vi "ivPIDantiWindup_Filter.vi"(4 "Saturation U":dbl, 6 "Saturation M":dbl, 7 "Reset":bool, 8 "PID Gains":cluster{"Kp":dbl, "Kd":dbl, "Ki":dbl, "Ts":dbl}={"Kp"=0.0, "Kd"=0.0, "Ki"=0.0, "Ts"=1.0}, 10 "Feedback":dbl, 11 "Reference":dbl) -> (3 "Control":dbl)   [LabVIEW 2016]
uses:
  <vilib>/ptbypt/NI_PtbyPt.lvlib
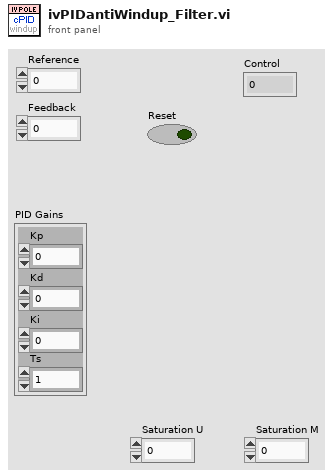
[diagram p1: front panel]
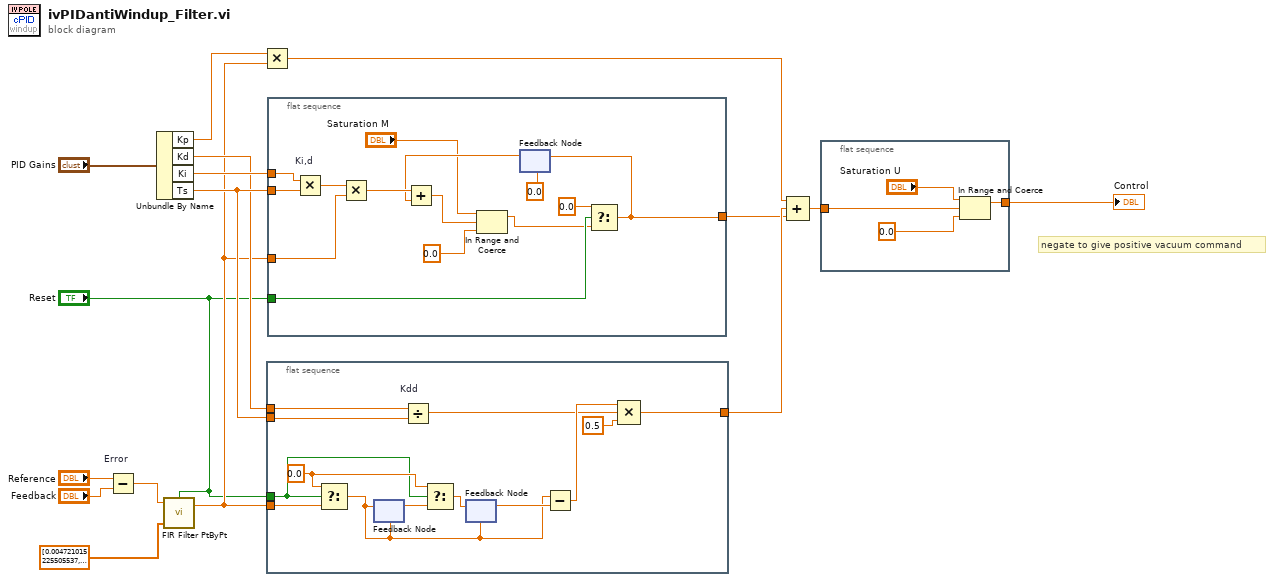
[diagram p0: block diagram]
diagram:
  # "negate to give positive vacuum command"
  n1 = Subtract "Error"(x="Reference", y="Feedback") -> (x-y=w3:dbl)
  n2 = Unbundle By Name("PID Gains") -> ("Kp"=w13:dbl, "Kd"=w7:dbl, "Ki"=w9:dbl, "Ts"=w8:dbl)
  n3 = call <vilib>:"FIR Filter PtByPt.vi"("initialize"="Reset", "Forward Coefficients"=dbl[] [0.004721015225505537, -0.000597520858147704, -0.0007222191680482241, -0.0009240752400420713, -0.0011718940020011637, -0.0014290675027618049, -0.001655610082476722, -0.001810828750726672, -0.0018564683384051574, -0.0017601113514815181, -0.0014985659826577272, -0.0010609475280570122, -0.00045115245663297467, 0.0003105570273631208, 0.0011870963911045983, 0.0021254013350882803, 0.003058653414690804, 0.003909870800248083, 0.004596736908457965, 0.005037430885863777, 0.005157124385221498, 0.0048947272089977295, 0.004209407822314554, 0.003086389589625448, 0.0015415339362916712, -0.000375730940404281, -0.002581493849840419, -0.004958699626008307, -0.007360845484991264, -0.009617979659942278, -0.01154478411206016, -0.012950365500293964, -0.013649238142369612, -0.013472870330683125, -0.012281090423405442, -0.009972618632918675, -0.006494008469075643, -0.0018463491181177501, 0.003910806096524346, 0.010658665773350283, 0.018221776192776273, 0.026373937065441805, 0.03484723658358649, 0.04334378220464025, 0.051549522736246536, 0.05914941116540325, 0.06584305682734187, 0.07135996753894874, 0.07547349129053045, 0.0780126331946144, 0.07887104290274363, 0.0780126331946144, 0.07547349129053045, 0.07135996753894874, 0.06584305682734187, 0.05914941116540325, 0.051549522736246536, 0.04334378220464025, 0.03484723658358649, 0.026373937065441805, 0.018221776192776273, 0.010658665773350283, 0.003910806096524346, -0.0018463491181177501, -0.006494008469075643, -0.009972618632918675, -0.012281090423405442, -0.013472870330683125, -0.013649238142369612, -0.012950365500293964, -0.01154478411206016, -0.009617979659942278, -0.007360845484991264, -0.004958699626008307, -0.002581493849840419, -0.000375730940404281, 0.0015415339362916712, 0.003086389589625448, 0.004209407822314554, 0.0048947272089977295, 0.005157124385221498, 0.005037430885863777, 0.004596736908457965, 0.003909870800248083, 0.003058653414690804, 0.0021254013350882803, 0.0011870963911045983, 0.0003105570273631208, -0.00045115245663297467, -0.0010609475280570122, -0.0014985659826577272, -0.0017601113514815181, -0.0018564683384051574, -0.001810828750726672, -0.001655610082476722, -0.0014290675027618049, -0.0011718940020011637, -0.0009240752400420713, -0.0007222191680482241, -0.000597520858147704, 0.004721015225505537] ("num_LP 2"), "x"=w3) -> ("Filtered x"=w4:dbl)  [unwired: 1 in, 1 out]
  n4 = Multiply(x=w13, y=w4) -> (x*y=w12:dbl)
  n5 = flat-sequence {
    tunnel: [w26] -> w11
    tunnel: w4 -> [w21]
    tunnel: w8 -> [w25]
    tunnel: w7 -> [w24]
    tunnel: "Reset" -> [w17]
    frame #0 {
      w18 = 0.0 ("t")
      n6 = Select(t=w18, s=w17, f=w21) -> (s? t:f=w22:dbl)
      n7 = feedback #1(w22) -> (w20:dbl)
      n8 = feedback-in #1(w22) -> ()
      n9 = Divide "Kdd"(x=w24, y=w25) -> (x/y=w23:dbl)
      n10 = Select(t=w18, s=w17, f=w20) -> (s? t:f=w19:dbl)
      n11 = feedback #2(w22) -> (w29:dbl)
      n12 = feedback-in #2(w19) -> ()
      n13 = Subtract(x=w22, y=w29) -> (x-y=w28:dbl)
      n14 = Compound Arithmetic op=MULTIPLY(w28, w23, 0.5 ("value")) -> (w26:dbl)
    }
  }
  n15 = flat-sequence {
    tunnel: [w32] -> w10
    tunnel: w4 -> [w43]
    tunnel: w9 -> [w41]
    tunnel: w8 -> [w39]
    tunnel: "Reset" -> [w35]
    frame #0 {
      n16 = Multiply "Ki,d"(x=w41, y=w39) -> (x*y=w40:dbl)
      n17 = Multiply(x=w40, y=w43) -> (x*y=w42:dbl)
      n18 = feedback #3(0.0 ("value")) -> (w36:dbl)
      n19 = Add(x=w42, y=w36) -> (x+y=w38:dbl)
      n20 = In Range and Coerce(upper limit="Saturation M", x=w38, lower limit=0.0 ("upper limit")) -> (coerced(x)=w34:dbl)  [unwired: 1 out]
      n21 = Select(t=0.0 ("value"), s=w35, f=w34) -> (s? t:f=w32:dbl)
      n22 = feedback-in #3(w32) -> ()
    }
  }
  n23 = Compound Arithmetic op=ADD(w12, w11, w10) -> (w6:dbl)
  n24 = flat-sequence {
    tunnel: w6 -> [w47]
    tunnel: [w46] -> w5
    frame #0 {
      n25 = In Range and Coerce(upper limit="Saturation U", x=w47, lower limit=0.0 ("upper limit")) -> (coerced(x)=w46:dbl)  [unwired: 1 out]
    }
  }
  "Control" <- w5
